vi "StrainPointGenerator.vi"(8 "error in (no error)":errorcluster, 11 "Strain Sweep Parameters":T1={"Max Motor Position"=1380.0, "# Intermediate Points"=5000, "Initial Direction"=enum."Tension"} {"# Intermediate Points" max=1390}) -> (0 "error out":errorcluster, 1 "Strain Points":dbl[](array[numeric]), 3 "Numer of Points":i32)   [LabVIEW 2014]
uses:
  <vilib>/measure/NI_MABase.lvlib
panel:
  out "Waveform Graph":dbl[](graph)
  # "LICENSED MATERIALS – PROPERTY OF IBM\nCopyright IBM Corp. 2016,\nALL RIGHTS RESERVED"
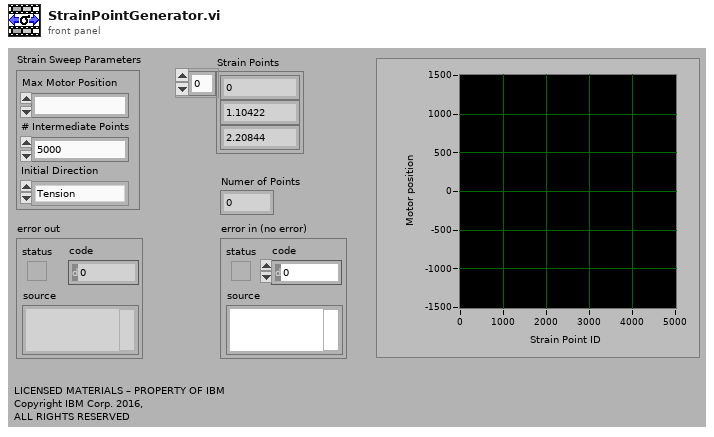
[diagram p1: front panel]
types:
  T1 = cluster{"Max Motor Position":ext, "# Intermediate Points":u32, "Initial Direction":enum16{"Tension", "Compression"}}
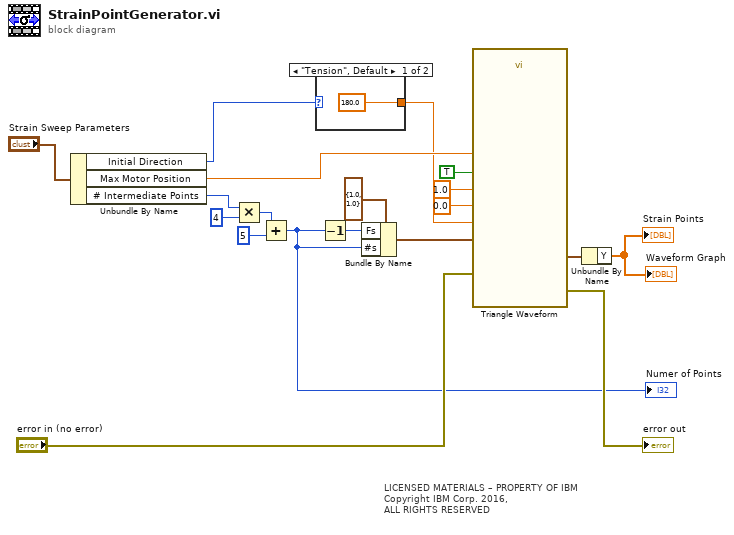
[diagram p0: block diagram]
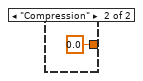
[diagram p2: hidden frame]
diagram:
  # "LICENSED MATERIALS – PROPERTY OF IBM\nCopyright IBM Corp. 2016,\nALL RIGHTS RESERVED"
  n1 = Unbundle By Name("Strain Sweep Parameters") -> ("Initial Direction"=w1:enum16{"Tension", "Compression"}, "Max Motor Position"=w8:ext, "# Intermediate Points"=w4:u32)
  n2 = Multiply(x=w4, y=u32 4) -> (x*y=w7:u32)
  n3 = Add(x=w7, y=u32 5) -> (x+y=w3:u32)
  "Numer of Points" <- w3
  n4 = case shown="\"Tension\", Default" w1 {
    tunnel: [180.0 ("offset") 0.0 ("offset")] -> w2
    frame "Tension", Default {
    }
    frame "Compression" {
    }
  }
  n5 = Decrement(x=w3) -> (x-1=w13:u32)
  n6 = Bundle By Name(cluster=cluster{"Fs":dbl, "#s":dbl} {"Fs"=1.0, "#s"=1.0} ("sampling info 2"), "Fs"=w13, "#s"=w3) -> (w15:cluster{"Fs":dbl, "#s":dbl})
  n7 = call <vilib>:"Triangle Waveform.vi"("offset"=0.0, "sampling info"=w15, "reset signal"=TRUE, "error in (no error)"="error in (no error)", "phase"=w2, "amplitude"=w8, "frequency"=1.0 ("Fs")) -> ("error out"=→"error out":errorcluster, "signal out"=w12:waveform(dbl))  [unwired: 3 out]
  n8 = Unbundle By Name(w12) -> ("Y"=→"Strain Points" →"Waveform Graph":dbl[])
